vi "AD（V1.0）.vi"() -> (1 "时域谱":dbl[](graph), 2 "幅频谱":dbl[](graph))   [LabVIEW 2018]
uses:
  <vilib>/Analysis/2dsp.llb/Real FFT.vi
  INF/amd64/PCI8502_32.dll
  <vilib>/Analysis/NI_AALPro.lvlib
panel:
  out "数值 2":i32
  out "数值":i32
  # "[220，2000]"
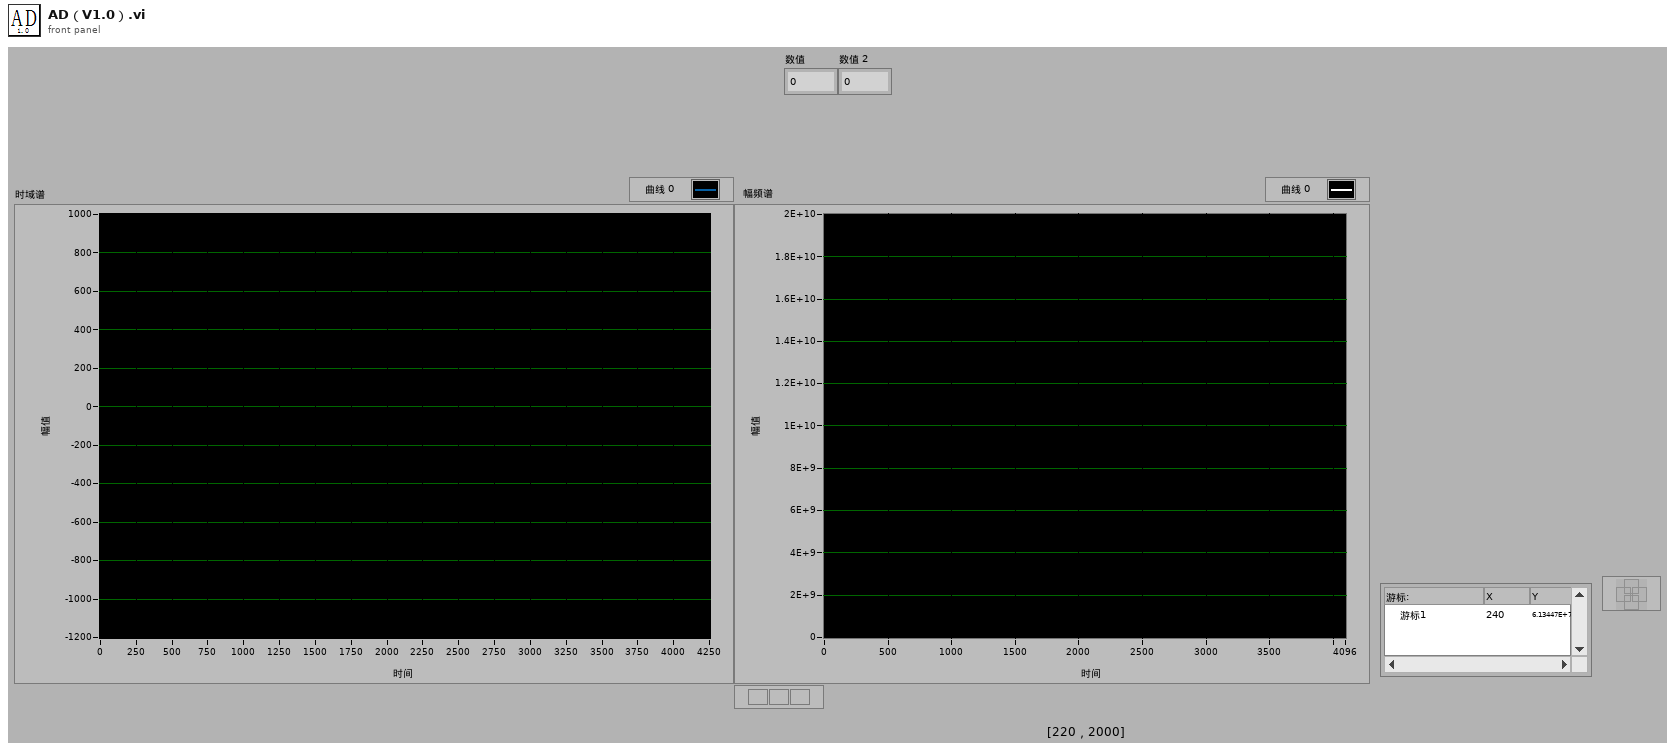
[diagram p1: front panel]
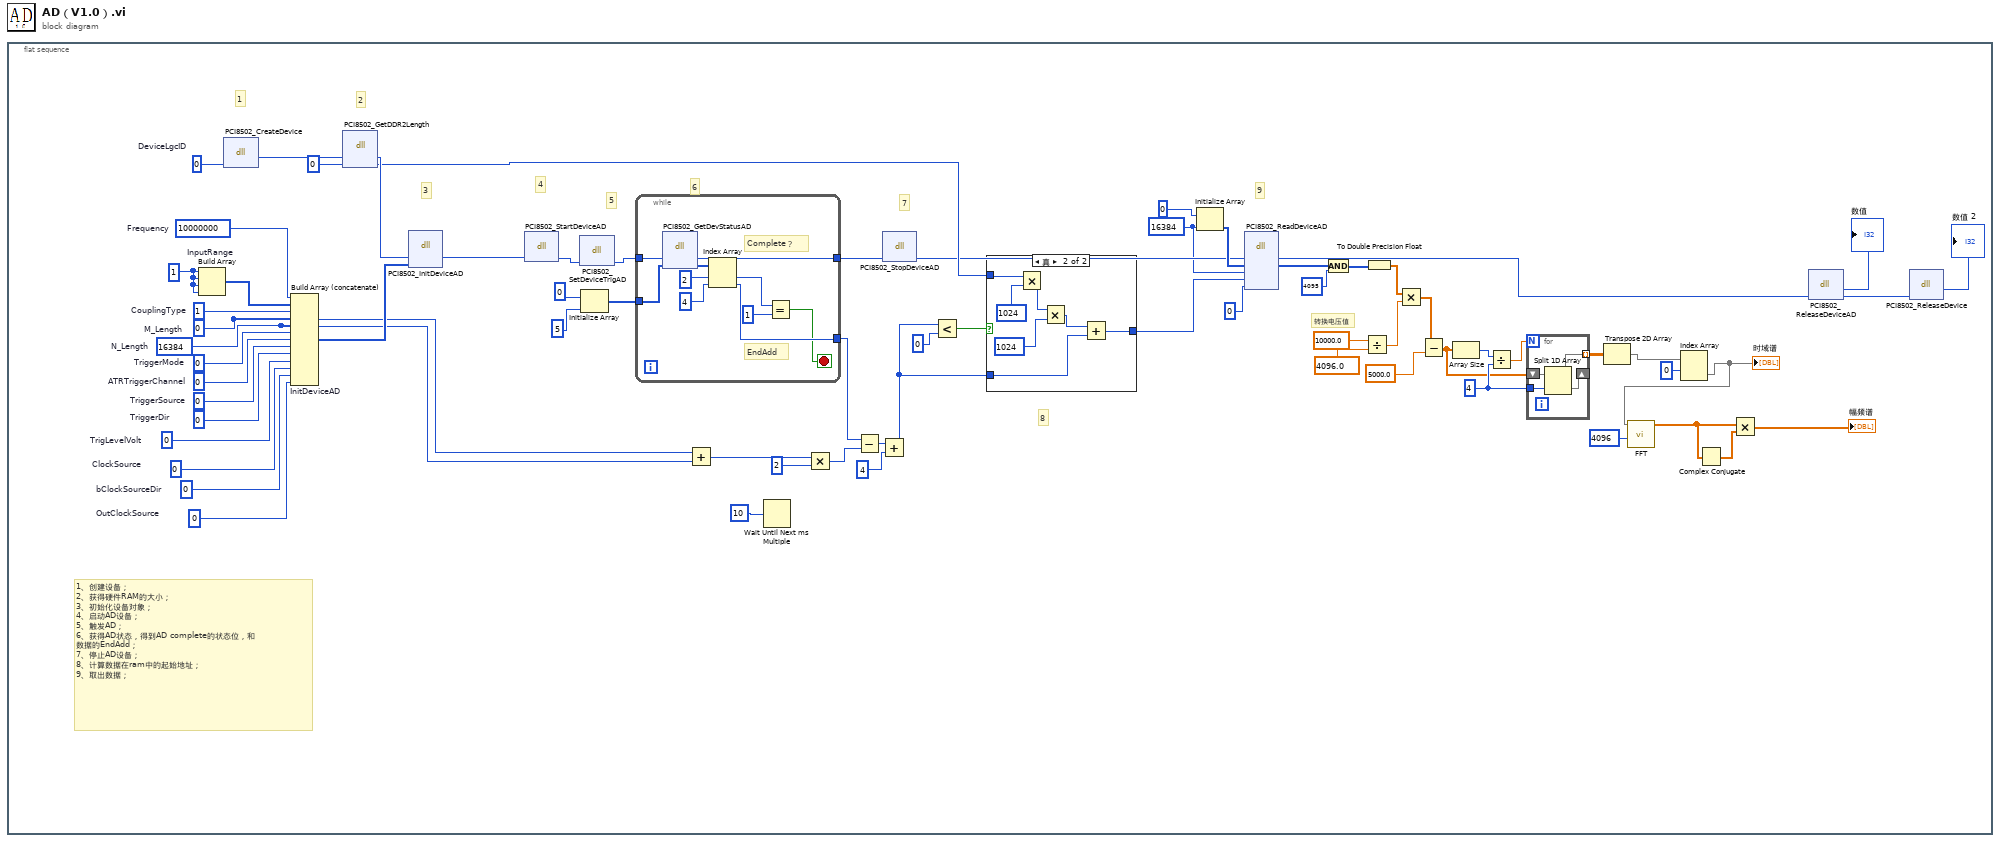
[diagram p0: block diagram]
diagram:
  n1 = flat-sequence {
    frame #0 {
      w16 = 4
      w18 = 16384 ("dimension size")
      w57 = 0  # OutClockSource
      w58 = 0  # bClockSourceDir
      w60 = 10000000  # Frequency
      w61 = 0  # ClockSource
      w62 = 0  # TrigLevelVolt
      w5 = 1
      w63 = 0  # TriggerDir
      w64 = 0  # TriggerSource
      w65 = 0  # ATRTriggerChannel
      w66 = 0  # TriggerMode
      w50 = 16384  # N_Length
      w51 = 0  # M_Length
      w67 = 1  # CouplingType
      w68 = 0  # DeviceLgcID
      # "9"
      # "8"
      # "7"
      # "6"
      # "5"
      # "4"
      # "转换电压值"
      # "1、创建设备；\n2、获得硬件RAM的大小；\n3、初始化设备对象；\n4、启动AD设备；\n5、触发AD；\n6、获得AD状态，得到AD complete的状态位，和\n数据的EndAdd；\n7、停止AD设备；\n8、计算数据在ram中的起始地址；\n9、取出数据；"
      # "3"
      # "2"
      # "1"
      n2 = Build Array "InputRange"(w5, w5, w5, w5) -> (w4:i32[])
      n3 = dll-call lib="PTH2abs CUsersBlueMessDesktopWork2020SAR ControllerSAR-Controller\treferencearté­ç¯æ«æç¨åºééå¡æ§å¶INFamd64\nPCI8502_32" fn="PCI8502_CreateDevice" label="CreateDevice"("DeviceLgcID"=w68) -> (w1:i32)  [unwired: 4 in, 2 out]
      n4 = Build Array (concatenate) "InitDeviceAD"(w60, w4, w67, w51, w50, w66, w65, w64, w63, w62, w61, w58, w57) -> (w59:i32[])
      n5 = dll-call lib="PTH2abs CUsersBlueMessDesktopWork2020SAR ControllerSAR-Controller\treferencearté­ç¯æ«æç¨åºééå¡æ§å¶INFamd64\nPCI8502_32" fn="PCI8502_GetDDR2Length" label="GetDDR2Length"("hDevice"=w1, "pulDDR2Length"=u32 0) -> ("hDevice"=w55:i32, "pulDDR2Length"=w53:u32)  [unwired: 4 in, 2 out]
      n6 = dll-call lib="PTH2abs CUsersBlueMessDesktopWork2020SAR ControllerSAR-Controller\treferencearté­ç¯æ«æç¨åºééå¡æ§å¶INFamd64\nPCI8502_32" fn="PCI8502_InitDeviceAD" label="InitDeviceAD"("hDevice"=w55, "pADPara"=w59) -> ("hDevice"=w56:i32)  [unwired: 5 in, 2 out]
      n7 = dll-call lib="PTH2abs CUsersBlueMessDesktopWork2020SAR ControllerSAR-Controller\treferencearté­ç¯æ«æç¨åºééå¡æ§å¶INFamd64\nPCI8502_32" fn="PCI8502_StartDeviceAD" label="StartDeviceAD"("hDevice"=w56) -> ("hDevice"=w48:i32)  [unwired: 4 in, 2 out]
      n8 = dll-call lib="PTH2abs CUsersBlueMessDesktopWork2020SAR ControllerSAR-Controller\treferencearté­ç¯æ«æç¨åºééå¡æ§å¶INFamd64\nPCI8502_32" fn="PCI8502_SetDeviceTrigAD" label="SetDeviceTrigAD"("hDevice"=w48) -> ("hDevice"=w25:i32)  [unwired: 4 in, 2 out]
      n9 = Initialize Array(0, 5) -> (w22:i32[])
      n10 = while {
        tunnel: [w77] -> w21
        tunnel: w25 -> [w76]
        tunnel: w22 -> [w75]
        tunnel: [w74] -> w19
        stop <- w73 stop-if-true
        # "EndAdd"
        # "Complete？"
        n11 = dll-call lib="PTH2abs CUsersBlueMessDesktopWork2020SAR ControllerSAR-Controller\treferencearté­ç¯æ«æç¨åºééå¡æ§å¶INFamd64\nPCI8502_32" fn="PCI8502_GetDevStatusAD" label="GetDevStatusAD"("hDevice"=w76, "pADStatus"=w75) -> ("hDevice"=w74:i32, "pADStatus"=w79:i32[])  [unwired: 4 in, 2 out]
        n12 = Index Array(array=w79, index #1=2, index #2=4) -> (element #1=w81:i32, element #2=w77:i32)
        n13 = Equal?(x=w81, y=1) -> (x = y?=w73:bool)
      }
      n14 = Add(x=w51, y=w50) -> (x+y=w20:i32)
      n15 = Wait Until Next ms Multiple(millisecond multiple=u32 10) -> ()  [unwired: 1 out]
      n16 = Multiply(x=w20, y=u32 2) -> (x*y=w33:u32)
      n17 = Subtract(x=w21, y=w33) -> (x-y=w35:u32)
      n18 = Add(x=w35, y=u32 4) -> (x+y=w30:u32)
      n19 = dll-call lib="PTH2abs CUsersBlueMessDesktopWork2020SAR ControllerSAR-Controller\treferencearté­ç¯æ«æç¨åºééå¡æ§å¶INFamd64\nPCI8502_32" fn="PCI8502_StopDeviceAD" label="StopDeviceAD"("hDevice"=w19) -> ("hDevice"=w36:i32)  [unwired: 4 in, 2 out]
      n20 = Less?(x=w30, y=u32 0) -> (x < y?=w26:bool)
      n21 = case shown="真" w26 {
        tunnel: w30 -> [w83 w86]
        tunnel: [w83 w85] -> w31
        tunnel: w53 -> [_ w84]
        frame False {
        }
        frame True {
          n22 = Multiply(x=w84, y=u32 1024) -> (x*y=w89:u32)
          n23 = Multiply(x=w89, y=u32 1024) -> (x*y=w87:u32)
          n24 = Add(x=w87, y=w86) -> (x+y=w85:u32)
        }
      }
      n25 = Initialize Array(0, w18) -> (w37:i32[])
      n26 = dll-call lib="PTH2abs CUsersBlueMessDesktopWork2020SAR ControllerSAR-Controller\treferencearté­ç¯æ«æç¨åºééå¡æ§å¶INFamd64\nPCI8502_32" fn="PCI8502_ReadDeviceAD" label="ReadDeviceAD"("hDevice"=w36, "ADBuffer"=w37, "nReadSizeWords"=w18, "ulStartAddr"=w31, "nRetSizeWords"=0) -> ("hDevice"=w49:i32, "ADBuffer"=w28:u16[])  [unwired: 7 in, 2 out]
      n27 = And(x=w28, y=4095) -> (x .and. y?=w39:i32[])
      n28 = Divide(x=10000.0, y=4096.0) -> (x/y=w41:dbl)
      n29 = To Double Precision Float(number=w39) -> (double precision float=w42:dbl[])
      n30 = Multiply(x=w42, y=w41) -> (x*y=w40:dbl[])
      n31 = Subtract(x=w40, y=5000.0) -> (x-y=w14:dbl[])
      n32 = Array Size(array=w14) -> (size(s)=w17:i32)
      n33 = Divide(x=w17, y=w16) -> (x/y=w15:dbl)
      n34 = for {
        N: w15 -> [_]
        tunnel: w16 -> [w72]
        shift-right: [w70] -> _
        shift-left: w14 -> [w71]
        tunnel: [w69] -> w13 mode=indexing
        n35 = Split 1D Array(array=w71, index=w72) -> (first subarray=w69:dbl[], second subarray=w70:dbl[])
      }
      n36 = Transpose 2D Array(2D array=w13) -> (transposed array=w11:dbl[][])
      n37 = Index Array(array=w11, index (row)=0 ("索引 (行)")) -> (element=w9:dbl[])  [unwired: 1 in]
      "时域谱" <- w9
      n38 = call-poly <vilib>:"FFT.vi"("FFT size"=4096 ("m"), "X"=w9) -> ("FFT {X}"=w8:cdb[])  [unwired: 8 in, 1 out]
      n39 = Complex Conjugate(1:w8) -> (0:w7:cdb[])
      n40 = Multiply(x=w8, y=w7) -> (x*y=→"幅频谱":cdb[])
      n41 = dll-call lib="PTH2abs CUsersBlueMessDesktopWork2020SAR ControllerSAR-Controller\treferencearté­ç¯æ«æç¨åºééå¡æ§å¶INFamd64\nPCI8502_32" fn="PCI8502_ReleaseDeviceAD" label="ReleaseDeviceAD"("hDevice"=w49) -> (→"数值":i32, "hDevice"=w52:i32)  [unwired: 3 in, 2 out]
      n42 = dll-call lib="PTH2abs CUsersBlueMessDesktopWork2020SAR ControllerSAR-Controller\treferencearté­ç¯æ«æç¨åºééå¡æ§å¶INFamd64\nPCI8502_32" fn="PCI8502_ReleaseDevice" label="ReleaseDevice"("hDevice"=w52) -> (→"数值 2":i32)  [unwired: 4 in, 2 out]
    }
  }
